vi "subFindMatchingDependencyType.vi"(11 "URL":string) -> (3 "Match?":bool)   [LabVIEW 2020, in "SolutionBuilder.lvlib" / "SolutionBuilder.lvclass"]
uses:
  SolutionBuilder/SolutionBuilder.lvclass
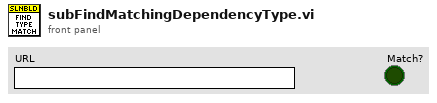
[diagram p1: front panel]
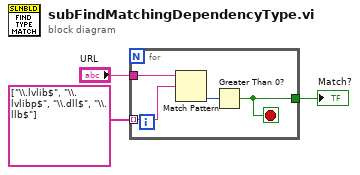
[diagram p0: block diagram]
diagram:
  n1 = for {
    tunnel: [w4] -> w3
    tunnel: "URL" -> [w6]
    tunnel: string[] ["\\.lvlib$", "\\.lvlibp$", "\\.dll$", "\\.llb$"] -> [w5] mode=indexing
    stop <- w4 stop-if-true
    n2 = Match Pattern(string=w6, regular expression=w5) -> (offset past match=w7:i32)  [unwired: 1 in, 3 out]
    n3 = Greater Than 0?(x=w7) -> (x > 0?=w4:bool)
  }
  "Match?" <- w3
